vi "Write FromFilePrefixCharacters.vi"(8 "error in (no error)":errorcluster, 10 "FromFilePrefixCharacters":string, 11 "ParserConfig in":refnum<class "ParserConfig.lvclass">) -> (0 "error out":errorcluster, 3 "ParserConfig out":refnum<class "ParserConfig.lvclass">)   [LabVIEW 2022 SP3, in "ArgumentParser.lvlib" / "ParserConfig.lvclass"]
uses:
  ParserConfig.lvclass
  ParserConfig.lvclass/ParserConfig.ctl
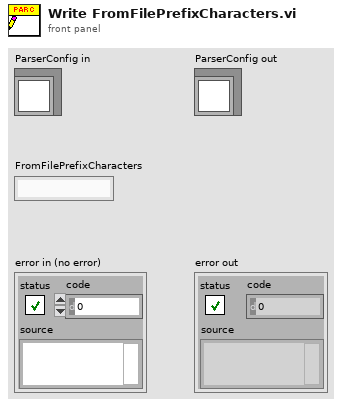
[diagram p1: front panel]
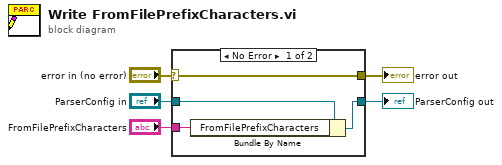
[diagram p0: block diagram]
diagram:
  n1 = case shown="No Error" "error in (no error)" {
    selector: "error in (no error)" -> [w9 w10]
    tunnel: [w9 w10] -> w4
    tunnel: [w7 w11] -> w2
    tunnel: "ParserConfig in" -> [w8 w11]
    tunnel: "FromFilePrefixCharacters" -> [w6 _]
    frame No Error {
      n2 = Bundle By Name(cluster=w8, "FromFilePrefixCharacters"=w6) -> (w7:refnum<class "ParserConfig.lvclass">)
    }
    frame Error {
    }
  }
  "error out" <- w4
  "ParserConfig out" <- w2
